vi "Sweeping Turn.vi"(5 "PID gains":T3={"proportional gain (Kc)"=0.01, "integral time (Ti, min)"=0.0, "derivative time (Td, min)"=0.0} {"derivative time (Td, min)" format="%.3f"; "integral time (Ti, min)" format="%.3f"; "proportional gain (Kc)" format="%.3f"}, 6 "Target Yaw":dbl, 8 "error in":errorcluster, 9 "Acceptable Range":dbl=5.0, 11 "PigeonIMUDevRef":T1={"DeviceStatus"={"status"=FALSE, "code"=0, "source"=""}, "Device Number"=2, "Type"=33554432, "Device ID"=33554434, "Handle"=42762848, "UsageFrame"=0, "Library Path"=path "libCTRE_PhoenixCCI.so"} {"Type" items=["CAN"=352321536, "TalonSRX"=33554432]}) -> (0 "error out":errorcluster, 2 "Yaw":dbl=90.0439453125, 3 "Yaw Output":dbl=0.075 format="%.2f", 4 "Stop":bool=TRUE)   [LabVIEW 2018]
uses:
  <vilib>/Rock Robotics/WPI/ThirdParty/Phoenix-LabVIEW/Pigeon IMU/CTRE_PigeonIMU_DeviceRef.ctl
  <vilib>/Rock Robotics/WPI/ThirdParty/Phoenix-LabVIEW/Pigeon IMU/CTRE_PigeonIMU_ConnectionType.ctl
  <vilib>/addons/control/pid/pid.llb/PID (DBL).vi
  <vilib>/addons/control/pid/NI_PID_pid.lvlib
panel:
  out "Target Yaw out":dbl=93.955078125
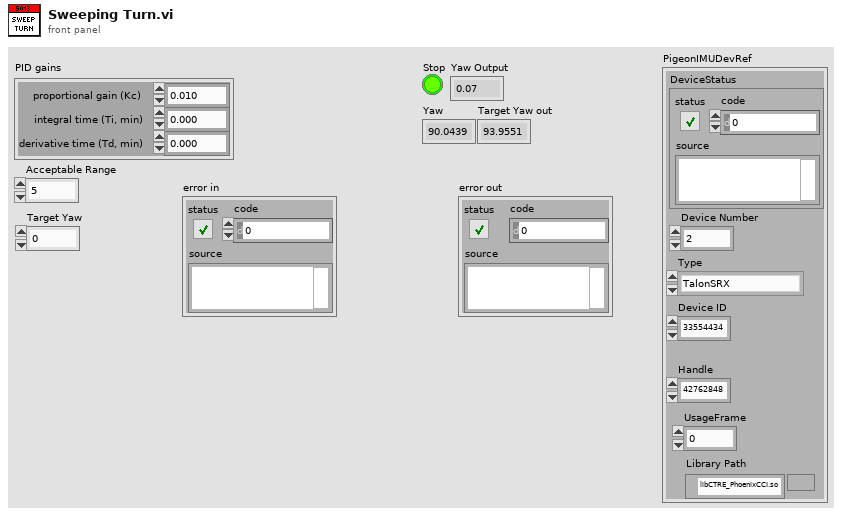
[diagram p1: front panel]
types:
  T1 = typedef "CTRE_PigeonIMU_DeviceRef.ctl" = cluster{"DeviceStatus":errorcluster, "Device Number":u8, "Type":T2, "Device ID":u32, "Handle":u64, "UsageFrame":u32, "Library Path":path}
  T2 = typedef "CTRE_PigeonIMU_ConnectionType.ctl" = u32
  T3 = cluster{"proportional gain (Kc)":dbl, "integral time (Ti, min)":dbl, "derivative time (Td, min)":dbl}
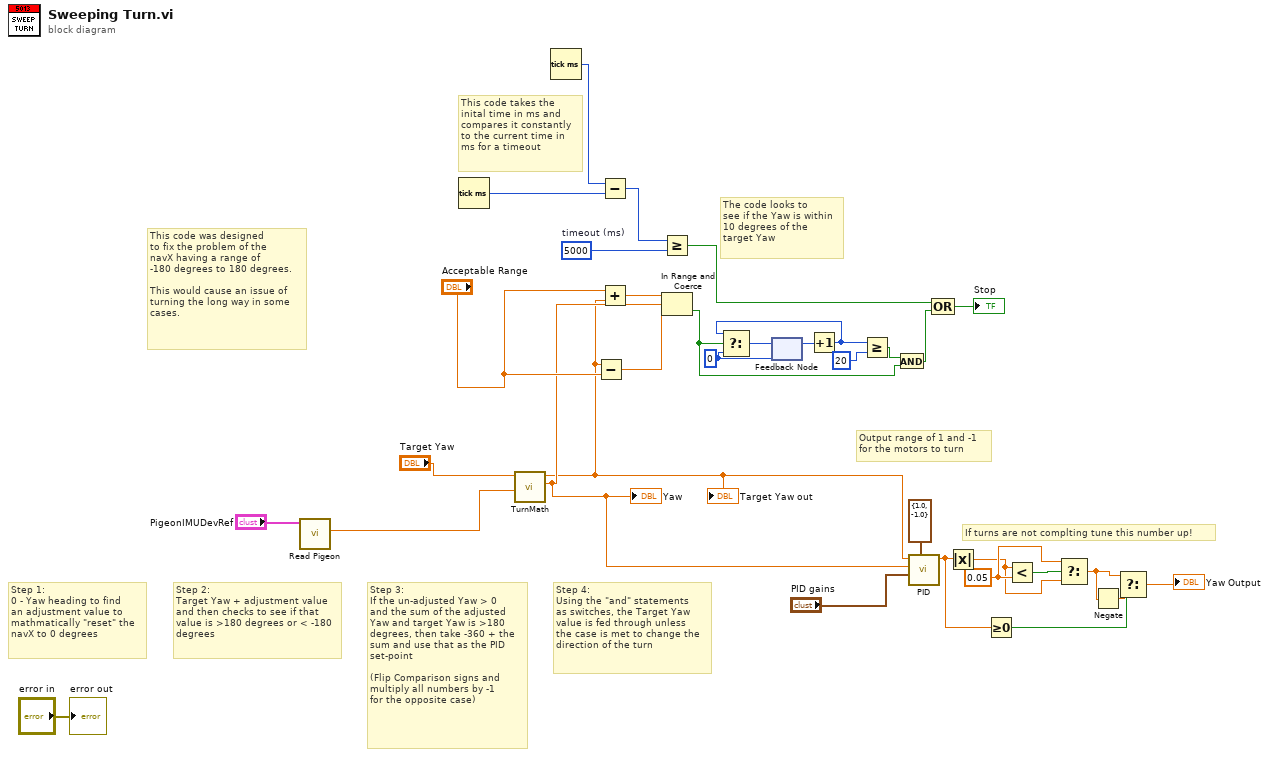
[diagram p0: block diagram]
diagram:
  w10 = 0
  w17 = 0.05 ("y")
  w25 = u32 5000  # timeout (ms)
  # "If turns are not complting tune this number up!"
  # "This code was designed\nto fix the problem of the\nnavX having a range of \n-180 degrees to 180 degrees.\n\nThis would cause an issue of\nturning the long way in some\ncases."
  # "Output range of 1 and -1\nfor the motors to turn"
  # "Step 4:\nUsing the \"and\" statements\nas switches, the Target Yaw\nvalue is fed through unless\nthe case is met to change the\ndirection of the turn"
  # "Step 3:\nIf the un-adjusted Yaw > 0 \nand the sum of the adjusted \nYaw and target Yaw is >180\ndegrees, then take -360 + the \nsum and use that as the PID \nset-point\n\n(Flip Comparison signs and\nmultiply all numbers by -1 \nfor the opposite case)"
  # "Step 2:\nTarget Yaw + adjustment value\nand then checks to see if that \nvalue is >180 degrees or < -180\ndegrees"
  # "Step 1: \n0 - Yaw heading to find\nan adjustment value to \nmathmatically \"reset\" the\nnavX to 0 degrees"
  # "The code looks to \nsee if the Yaw is within\n10 degrees of the \ntarget Yaw"
  # "This code takes the\ninital time in ms and\ncompares it constantly\nto the current time in\nms for a timeout"
  n1 = call "Read Pigeon.vi"("PigeonIMUDevRef"="PigeonIMUDevRef") -> ("Yaw"=w1:dbl)  [unwired: 10 in]
  n2 = Tick Count (ms)() -> (millisecond timer value=w32:u32)
  n3 = call "TurnMath.vi"("Yaw in"=w1, "Target Yaw in"="Target Yaw") -> ("Yaw out"=w20:dbl, "Target Yaw out"=w19:dbl)  [unwired: 8 in]
  "Yaw" <- w20
  "Target Yaw out" <- w19
  n4 = Tick Count (ms)() -> (millisecond timer value=w29:u32)
  n5 = Subtract(x=w19, y="Acceptable Range") -> (x-y=w24:dbl)
  n6 = Subtract(x=w29, y=w32) -> (x-y=w28:u32)
  n7 = Add(x="Acceptable Range", y=w19) -> (x+y=w23:dbl)
  n8 = Greater Or Equal?(x=w28, y=w25) -> (x >= y?=w26:bool)
  n9 = In Range and Coerce(upper limit=w23, x=w20, lower limit=w24) -> (In Range?=w4:bool)  [unwired: 1 out]
  n10 = feedback #1(w10) -> (w9:i32)
  n11 = Increment(x=w9) -> (x+1=w8:i32)
  n12 = Select(t=w8, s=w4, f=w10) -> (s? t:f=w7:i32)
  n13 = feedback-in #1(w7) -> ()
  n14 = Greater Or Equal?(x=w8, y=20) -> (x >= y?=w6:bool)
  n15 = And(x=w6, y=w4) -> (x .and. y?=w5:bool)
  n16 = call-poly <vilib>:"PID.vi"("output range"=cluster{"output high":dbl, "output low":dbl} {"output high"=1.0, "output low"=-1.0}, "PID gains"="PID gains", "process variable"=w20, "setpoint"=w19) -> ("output"=w15:dbl)  [unwired: 6 in, 1 out]
  n17 = Compound Arithmetic op=OR(w26, w5) -> (→"Stop":bool)
  n18 = Absolute Value(x=w15) -> (abs(x)=w16:dbl)
  n19 = Greater Or Equal To 0?(x=w15) -> (x >= 0?=w14:bool)
  n20 = Less?(x=w16, y=w17) -> (x < y?=w18:bool)
  n21 = Select(t=w17, s=w18, f=w16) -> (s? t:f=w12:dbl)
  n22 = Negate(x=w12) -> (-x=w13:dbl)
  n23 = Select(t=w12, s=w14, f=w13) -> (s? t:f=→"Yaw Output":dbl)
  "error out" <- "error in"
